vi "Open_ExcelApp.vi"(0 "excel是否可见":bool, 1 "错误输入（无错误）":errorcluster) -> (2 "application引用":refnum<k7>, 3 "documentl引用":refnum<k7>, 4 "错误输出":errorcluster)   [LabVIEW 2014]
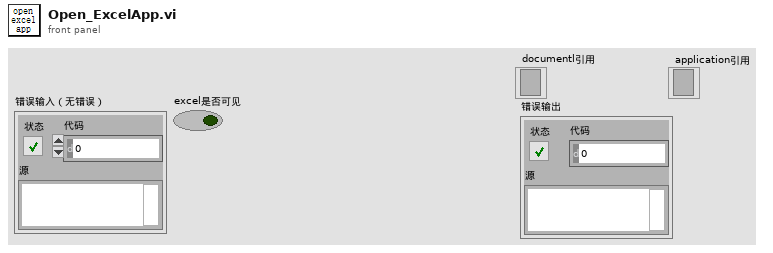
[diagram p1: front panel]
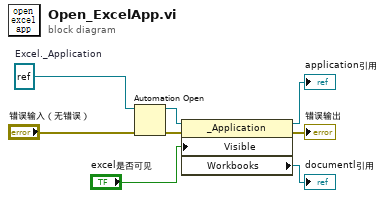
[diagram p0: block diagram]
diagram:
  w8 = refnum<k7> refnum  # Excel._Application
  n1 = Automation Open(error in (no error)="错误输入（无错误）", Automation Refnum=w8) -> (Automation Refnum=w5:refnum<k7>, error out=w4:errorcluster)  [unwired: 2 in]
  n2 = property class="_Application"(reference=w5, error in=w4, "Visible"="excel是否可见") -> (reference out=→"application引用":refnum<k7>, error out=→"错误输出":errorcluster, "Workbooks"=→"documentl引用":refnum<k7>)
